vi "Initialize Lasers.vi"(8 "error in (no error)":errorcluster, 11 "Application in":refnum<class "Application.lvclass">) -> (0 "error out":errorcluster, 3 "Application out":refnum<class "Application.lvclass">)   [LabVIEW 2018, in "Application.lvlib" / "Application.lvclass"]
uses:
  Application.lvclass
  C:/Program Files/National Instruments/LabVIEW 2018/vi.lib/ActorFramework/Actor/Actor.lvclass
  Hardware/Laser Quantum/Laser Quantum.lvclass
  Application.lvclass/Application.ctl
  <vilib>/ActorFramework/Actor/Actor.lvclass
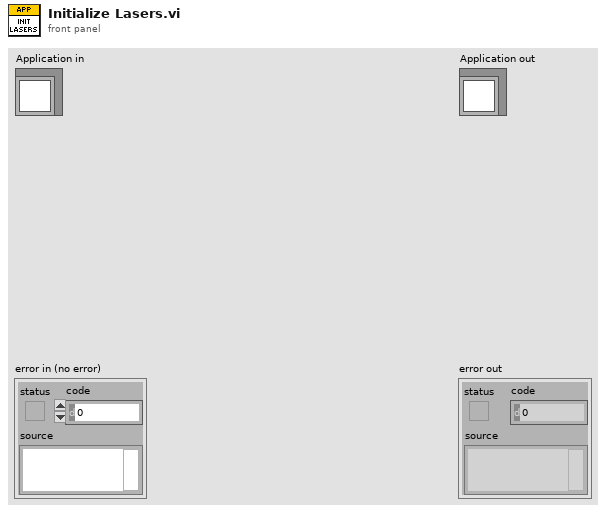
[diagram p1: front panel]
types:
  T1 = typedef "Laser Configuration.ctl" = cluster{"Excitation":T2, "Serial Port":refnum<visa-resource-name>, "Laser Type":enum16{"Disable", "Laser Quantum", "Coherent OBIS", "PRM1-Z8"}, "Polarizer Amplitude":dbl, "Polarizer Theta Zero":dbl}
  T2 = typedef "Excitation.ctl" = enum16{"Cy2 (473 nm)", "Cy3 (532 nm)", "Cy5 (639 nm)", "Cy7 (730 nm)", "Cy2/Cy3", "Cy3/Cy5", "Cy3/Cy7", "Cy5/Cy7"}
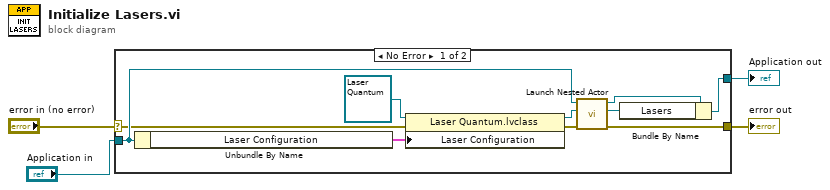
[diagram p0: block diagram]
diagram:
  n1 = case shown="No Error" "error in (no error)" {
    selector: "error in (no error)" -> [w5 w16]
    tunnel: [w6 w16] -> w3
    tunnel: [w7 w15] -> w1
    tunnel: "Application in" -> [w14 w15]
    frame No Error {
      n2 = Unbundle By Name(w14) -> ("Laser Configuration"=w10:T1[])
      n3 = property class="Laser Quantum.lvclass"(reference=refnum<class "Laser Quantum.lvclass"> refnum ("Laser Quantum.lvlib:Laser Quantum.lvclass"), error in=w5, "Laser Configuration"=w10) -> (reference out=w12:refnum<class "Laser Quantum.lvclass">, error out=w11:errorcluster)
      n4 = call <vilib>:"Launch Nested Actor.vi"("error in (no error)"=w11, "Nested Actor"=w12, "Caller Actor in"=w14) -> ("error out"=w6:errorcluster, "Nested Actor's Enqueuer"=w8:refnum<class "Message Enqueuer.lvclass">, "Caller Actor out"=w9:refnum<class "Application.lvclass">)  [unwired: 6 in]
      n5 = Bundle By Name(cluster=w9, "Lasers"=w8) -> (w7:refnum<class "Application.lvclass">)
    }
    frame Error {
    }
  }
  "error out" <- w3
  "Application out" <- w1
